vi "State data Look up float key.vi"(6 "Error on not found (T)":bool=TRUE, 7 "Key [string/enum]":variant, 8 "error in (no error)":errorcluster, 10 "Value if not found (0)":dbl, 11 "Fiber Auto Collimation state data in":refnum<class "Fiber Auto Collimation state data.lvclass">) -> (0 "error out":errorcluster, 1 "float Key found":bool, 2 "Float Key Value":dbl, 3 "Fiber Auto Collimation state data out":refnum<class "Fiber Auto Collimation state data.lvclass">)   [LabVIEW 2018, in "Fiber Auto Collimation state data.lvclass"]
doc: "Serial number of the Device Under Test."
uses:
  Fiber Auto Collimation state data.lvclass
  Fiber Auto Collimation state data.lvclass/Fiber Auto Collimation state data.ctl
  <userlib>/Recipe/Test Recipe classes/Test Recipe.lvclass
  C:/Program Files (x86)/National Instruments/LabVIEW 2018/user.lib/Recipe/nLight Recipe/nLight Recipe.lvclass
  <userlib>/Recipe/nLight Recipe/nLight Recipe.lvclass
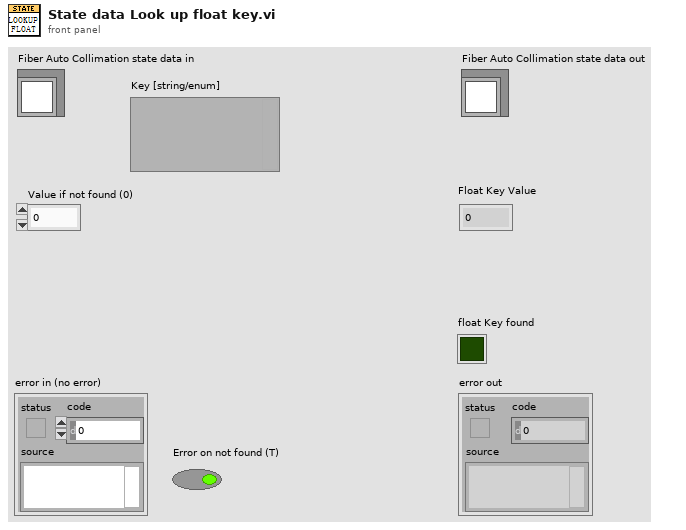
[diagram p1: front panel]
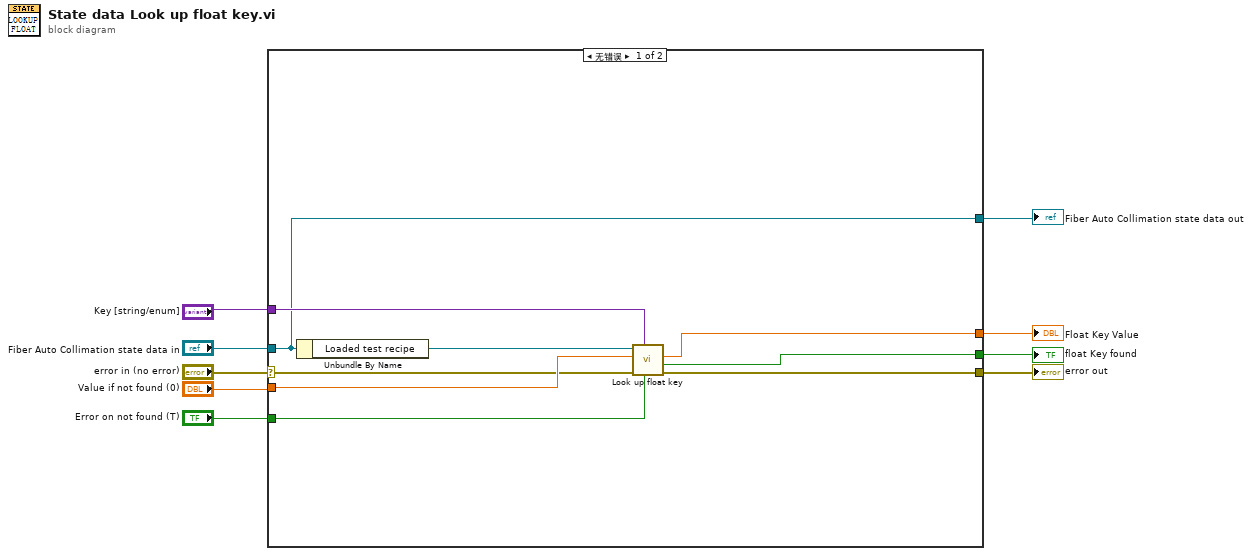
[diagram p0: block diagram]
diagram:
  n1 = case shown="无错误" "error in (no error)" {
    selector: "error in (no error)" -> [w15 w20]
    tunnel: [w13 w20] -> w8
    tunnel: [w10 w19] -> w1
    tunnel: "Fiber Auto Collimation state data in" -> [w10 w19]
    tunnel: "Key [string/enum]" -> [w17 _]
    tunnel: "Error on not found (T)" -> [w14 _]
    tunnel: [w12 _] -> w3
    tunnel: [w11 _] -> w5
    tunnel: "Value if not found (0)" -> [w16 _]
    frame No Error {
      n2 = Unbundle By Name(w10) -> ("Loaded test recipe"=w18:refnum<class "Test Recipe.lvclass">)
      n3 = call <userlib>:"Look up float key.vi"("Error on not found (T)"=w14, "Key [string/enum]"=w17, "error in (no error)"=w15, "Value if not found (0)"=w16, "nLight Recipe in"=w18) -> ("error out"=w13:errorcluster, "Float Key found"=w11:bool, "Float Key Value"=w12:dbl)  [unwired: 3 in, 1 out]
    }
    frame Error {
    }
  }
  "Fiber Auto Collimation state data out" <- w1
  "error out" <- w8
  "float Key found" <- w5
  "Float Key Value" <- w3
